vi "OCT with WavePond Clock.vi"() -> ()   [LabVIEW 2014]
doc: "I. Description:\nThis example demonstrates how to acquire a continuous amount of data (Waveform) using the DAQ device's internal clock.\n\nII. Instructions for Running:\n1. Create an analog input voltage channel.\n2. Set the rate for the sample clock. Additionally, define the sample mode to be continuous.\n3. Call the Start VI to start the acquisition.\n4. Read the waveform data in a loop until the user hits the stop button or an error occurs.\nNote: This example reads data from one or more channels and returns an array of data. Use the Index Array function to access an individual channel of data.\n5. Call the Clear Task VI to clear the Task.\n6. Use the popup dialog box to display an error if any.\n\nIV. I/O Connections Overview:\nMake sure your signal input terminal matches the Physical Channel I/O Control. For further connection information, refer to your hardware reference manual."
uses:
  ATS-VI/ATS_ctl/Device_Ctrl.ctl
  ATS-VI/ATS_ctl/ATS_Async_Ctrl.ctl
  ATS-VI/ATS_ctl/ATS_Async_Mode.ctl
  ATS-VI/ATS_ctl/ATS_DMA_Channel.ctl
  ATS-VI/ATS_ctl/ATS_ReadSamples.ctl
  ATS-VI/ATS_ctl/ATS_Check_Ctrl.ctl
  ATS-VI/ATS_ctl/ClockSource.ctl
  Galvo VIs/galvo_states.ctl
  Signal Processing/processing_states.ctl
  En Face/En Face States.ctl
  Saving Data/Saving Data States.ctl
  Type Defs/OCT Hardware States.ctl
  ATS-VI/ATS_ctl/Range.ctl
  ATS-VI/ATS_ctl/Impedance.ctl
  Type Defs/OCT Imaging Parameters Cluster.ctl
  Signal Processing/Display Raw Data states.ctl
  ATS-VI/ATS_ctl/ATS_Spec_Selector.ctl
  Classes/Galvo/Scanning Cluster.ctl
  Classes/Galvo/Galvo.lvclass
  Type Defs/OCT DAQ Channel Data Type.ctl
  Type Defs/Display States.ctl
  ATS-VI/ATS_ctl/Coupling.ctl
  ATS-VI/ATS_ctl/Bandwidth.ctl
  ATS-VI/ATS_ctl/InputCtrl.ctl
  ATS-VI/ATS_ctl/TriggerEngine.ctl
  ATS-VI/ATS_ctl/ExtTrigRange.ctl
  ATS-VI/ATS_ctl/ExtTrigger.ctl
  ATS-VI/ATS_ctl/TriggerOperation.ctl
  ATS-VI/ATS_ctl/Trigger.ctl
  ATS-VI/ATS_ctl/ClockRate.ctl
  ATS-VI/ATS_ctl/ClockEdge.ctl
  ATS-VI/ATS_ctl/Clock.ctl
  ATS-VI/ATS_ctl/Record.ctl
  ATS-VI/ATS_ctl/ATS_Global.ctl
  ATS-VI/ATS_ctl/ATS_Async_Status.ctl
  En Face/En Face Depth Parameters.ctl
  ATS-VI/ATS_ctl/ATS_Async_Setting.ctl
panel:
  in  "update en face image?":bool
  out "First Time?":bool
  out "Save Data":bool
  in  "Async_Setting":T1
  out "Processing Finished":bool
  in  "OCT Hardware States":T2=enum."Save Sweep"
  out "Save State":T3=enum."Initialize"
  out "Clock Length":u32=6304
  out "Reset DAQ":bool
  in  "Tab Control":T4(tab)
  in  "B-Scans Per Buffer":i32=1
  out "Async_Status":T5
  out "Current State":T2=enum."Set Resampling Array"
  in  "Channels":tag="Dev1/ao0:1"
  in  "Trigger Source":tag="/Dev1/PFI7"
  in  "Imaging Parameters":T6={"Points Per A-Scan"=0, "A-Scans per B-Scan"=0, "Voltage Range"=1.0, "Card Resolution (bits)"=12}
  in  "Setup_In":T7={"Record"={"Count"=1, "Presize"=0, "Length"=1408}, "Clock"={"ClckSource"=enum."External", "ClckRate"=17, "ClckEdge"=0, "Decimation"=0}, "Input A"={"Coupling"=enum."DC", "Range"=3, "Impedance"=enum."50 ohms", "Bandwidth"=enum."Full Bandwidth"}, "Input B"={"Coupling"=enum."DC", "Range"=3, "Impedance"=enum."50 ohms", "Bandwidth"=enum."Full Bandwidth"}, "Trigger"={"TrigOperation"=enum."Only X", "Timeout (s)"=1.0, "Trig. Delay"=0, "Engine X"={"Source"=enum."External", "Slope"=enum."Positive", "Level"=150}, "Engine Y"={"Source"=enum."Disable", "Slope"=enum."Positive", "Level"=128}, "ExtTrigControl"={"Coupling"=enum."DC", "Range"=enum."TTL"}}} {"Clock"."ClckEdge" items=["Rising", "Falling"]; "Clock"."ClckRate" items=["1 kS/s", "2 kS/s", "5 kS/s", "10 kS/s", "20 kS/s", "50 kS/s", "100 kS/s", "200 kS/s", "500 kS/s", "1 MS/s", "2 MS/s", "5 MS/s", "10 MS/s", "20 MS/s", "50 MS/s", "100 MS/s", "125 MS/s", "160 MS/s", "180 MS/s"]; "Input B"."Range" items=["200mV", "400mV", "800mV", "2 V", "4 V", "8 V", "16 V"]; "Trigger"."Timeout (s)" format="%.2f"; "Input A"."Range" items=["200mV", "400mV", "800mV", "2 V", "4 V", "8 V", "16 V"]}
  in  "OK Button":bool
  in  "Data Format":T23
  out "Channel A or B Phase (or Channel B Raw)":sgl[][](graph)
  out "Channel A or B Intensity (or Channel A Raw)":sgl[][](graph)
  in  "Display":T24
  out "En Face":dbl[][](graph)
  in  "En Face Parameters":T25={"En Face Start\nDepth"=50, "En Face End\nDepth"=200}
  in  "Save Sweep":bool
  in  "Scanning":T26={"Fast Axis Offset"=300.0, "Slow Axis Offset"=300.0, "Slow Axis Amp"=4.0, "Fast Axis Amp"=4.0, "Scan Pattern"=enum."Raster"} {"Fast Axis Amp" max=20 format="%#.2f"; "Slow Axis Amp" max=20 format="%#.2f"; "Slow Axis Offset" max=10 format="%#.2f"; "Fast Axis Offset" max=10 format="%#.2f"}
  in  "Stop Button":bool
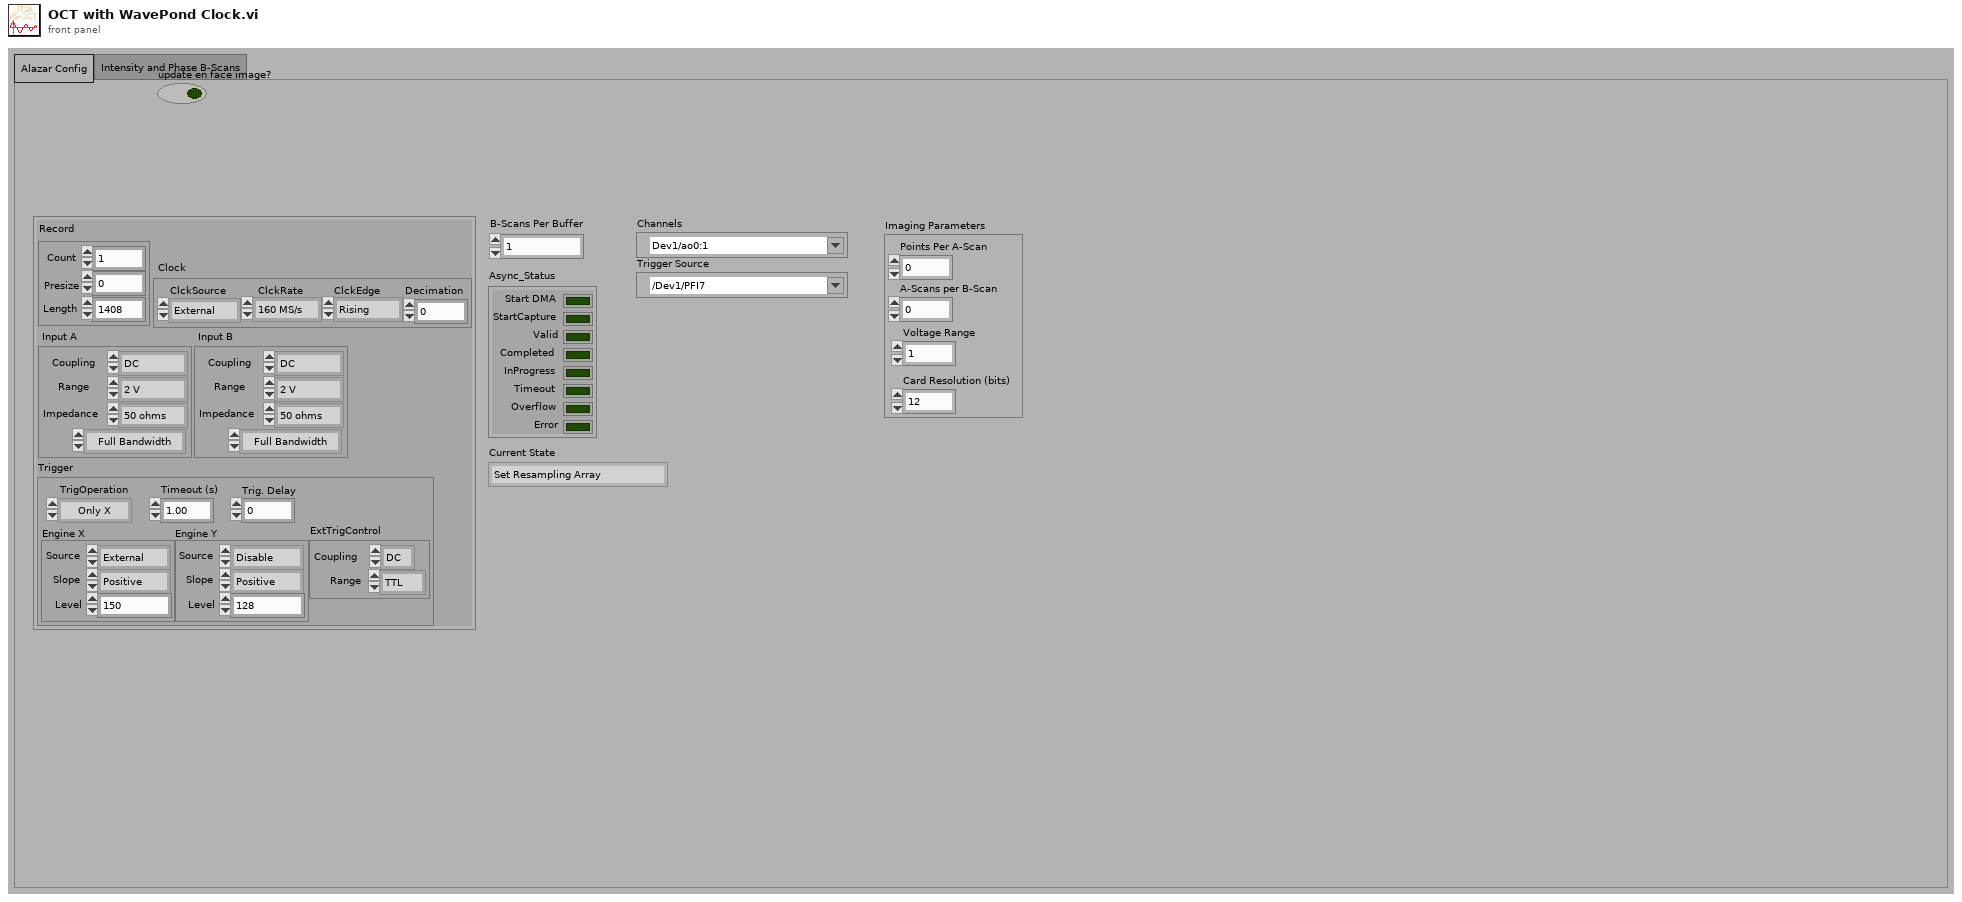
[diagram p1: front panel]
types:
  T1 = typedef "ATS_Async_Setting.ctl" = cluster{"UseHeader":u32, "Rec/Buffer":u32, "Total_Rec":u32, "DataBuffer":bool, "GetProcessedData":bool}
  T2 = typedef "OCT Hardware States.ctl" = enum16{"Acquire Data", "Initialize Laser", "Initialize Galvos", "Startup", "Reset DAQ", "Background Subtraction", "Acquire Background", "Update DAQ Parameters", "Stop", "Set Clock", "Initialize DAQ", "Set Resampling Array", "Save Sweep", "Configure Laser", "128 x 128", "512 x 512", "Review Data"}
  T3 = typedef "Saving Data States.ctl" = enum16{"Get Queue Size", "Get Queue", "Get Timeout", "Flush Queue", "Close Files", "Create Files", "Do Nothing", "Initialize", "Enqueue Data", "Save Data", "Shutdown"}
  T4 = enum32{"Alazar Config", "Intensity and Phase B-Scans"}
  T5 = typedef "ATS_Async_Status.ctl" = cluster{"Start DMA":bool, "StartCapture":bool, "Valid":bool, "Completed":bool, "InProgress":bool, "Timeout":bool, "Overflow":bool, "Error":bool}
  T6 = typedef "OCT Imaging Parameters Cluster.ctl" = cluster{"Points Per A-Scan":i32, "A-Scans per B-Scan":i32, "Voltage Range":sgl, "Card Resolution (bits)":u16}
  T7 = typedef "ATS_Global.ctl" = cluster{"Record":T8, "Clock":T9, "Input A":T13, "Input B":T13, "Trigger":T18}
  T8 = typedef "Record.ctl" = cluster{"Count":u32, "Presize":u32, "Length":u32}
  T9 = typedef "Clock.ctl" = cluster{"ClckSource":T10, "ClckRate":T11, "ClckEdge":T12, "Decimation":u32}
  T10 = typedef "ClockSource.ctl" = enum16{"Internal", "External", "Medium Ext.", "Slow Ext.", "Ext. AC", "Ext. DC", "Ext. (PLL)"}
  T11 = typedef "ClockRate.ctl" = u32
  T12 = typedef "ClockEdge.ctl" = u16
  T13 = typedef "InputCtrl.ctl" = cluster{"Coupling":T14, "Range":T15, "Impedance":T16, "Bandwidth":T17}
  T14 = typedef "Coupling.ctl" = enum16{"AC", "DC"}
  T15 = typedef "Range.ctl" = u32
  T16 = typedef "Impedance.ctl" = enum16{"1M ohms", "50 ohms"}
  T17 = typedef "Bandwidth.ctl" = enum16{"Full Bandwidth", "Reduce Bandwidth"}
  T18 = typedef "Trigger.ctl" = cluster{"TrigOperation":T19, "Timeout (s)":dbl, "Trig. Delay":u32, "Engine X":T20, "Engine Y":T20, "ExtTrigControl":T21}
  T19 = typedef "TriggerOperation.ctl" = enum16{"Only X", "Only Y", "X or Y", "X and Y", "X xor Y", "X and not Y", "not X and Y"}
  T20 = typedef "TriggerEngine.ctl" = cluster{"Source":enum32{"Chan_A", "Chan_B", "External", "Disable"}, "Slope":enum32{"Positive", "Negative"}, "Level":u32}
  T21 = typedef "ExtTrigger.ctl" = cluster{"Coupling":T14, "Range":T22}
  T22 = typedef "ExtTrigRange.ctl" = enum16{"1 V", "5 V", "TTL"}
  T23 = typedef "OCT DAQ Channel Data Type.ctl" = enum16{"Channel 1", "Channel 2", "Channel 1 and 2"}
  T24 = typedef "Display States.ctl" = enum16{"Channel A", "Channel B"}
  T25 = typedef "En Face Depth Parameters.ctl" = cluster{"En Face Start\nDepth":i32, "En Face End\nDepth":i32}
  T26 = typedef "Galvo.lvclass/Scanning Cluster.ctl" = cluster{"Fast Axis Offset":sgl, "Slow Axis Offset":sgl, "Slow Axis Amp":sgl, "Fast Axis Amp":sgl, "Scan Pattern":enum16{"Raster"}}
  T27 = typedef "ATS_Check_Ctrl.ctl" = enum16{"None", "NO_ATS9462", "ATS9462_Traditional", "Verify Board", "OnBoard Memory", "Board & Memory", "Master/Slave", "NO Master/Slave"}
  T28 = typedef "Device_Ctrl.ctl" = enum16{"Status", "About", "Arm", "ForceTrig", "Abort", "Initialize", "Init (NoPreset)", "Info", "Close", "Calibrate", "SetManually", "LED_ON", "LED_OFF"}
  T29 = typedef "ATS_Spec_Selector.ctl" = enum16{"None", "ClckSource", "ClckEdge", "ClckRate", "InputRange", "InputCoupling", "Impedance", "Bandwidth", "AsyncDMA", "Memory", "ExtTrigCoupling", "ExtTrigRange", "AUX_IO_Trig", "AUX_IO_Slope", "Trigger_Source"}
  T30 = typedef "galvo_states.ctl" = enum16{"Reset", "Reset Galvos?", "Center Galvos", "Register Callback", "Get Scan Parameters", "Show", "Initialize", "Run Raster", "Load Raster", "Run Circle", "Shutdown"}
  T31 = typedef "processing_states.ctl" = enum16{"Initialize", "Set Background", "Update Imaging Parameters", "Get Queue", "Process Data", "Get Size", "Flush Data", "Set Reample Array", "Get Last Processed BScan", "Shutdown"}
  T32 = typedef "Display Raw Data states.ctl" = enum16{"Add Raw", "Add Processed", "Show"}
  T33 = typedef "En Face States.ctl" = enum16{"Save BMP", "Show", "Clear En Face", "Update EnFace"}
  T34 = typedef "Processed OCT Data.ctl" = cluster{"Intensity A":sgl[][][], "Phase A":sgl[][][], "Intensity B":sgl[][][], "Phase B":sgl[][][]}
  T35 = enum8{"Enabled", "Disabled", "Disabled and Grayed Out"}
  T36 = typedef "ATS_Async_Ctrl.ctl" = enum16{"SetupDMA", "StartCapture", "Get", "Get_Stream", "Abort", "Stop"}
  T37 = typedef "ATS_ReadSamples.ctl" = cluster{"Offset":i32, "Length":u32}
  T38 = typedef "ATS_DMA_Channel.ctl" = enum16{"Channel_A", "Channel_B", "A & B"}
  T39 = typedef "ATS_Async_Mode.ctl" = enum16{"Continuous", "Triggered", "No-Pre-Trigger", "Traditional"}
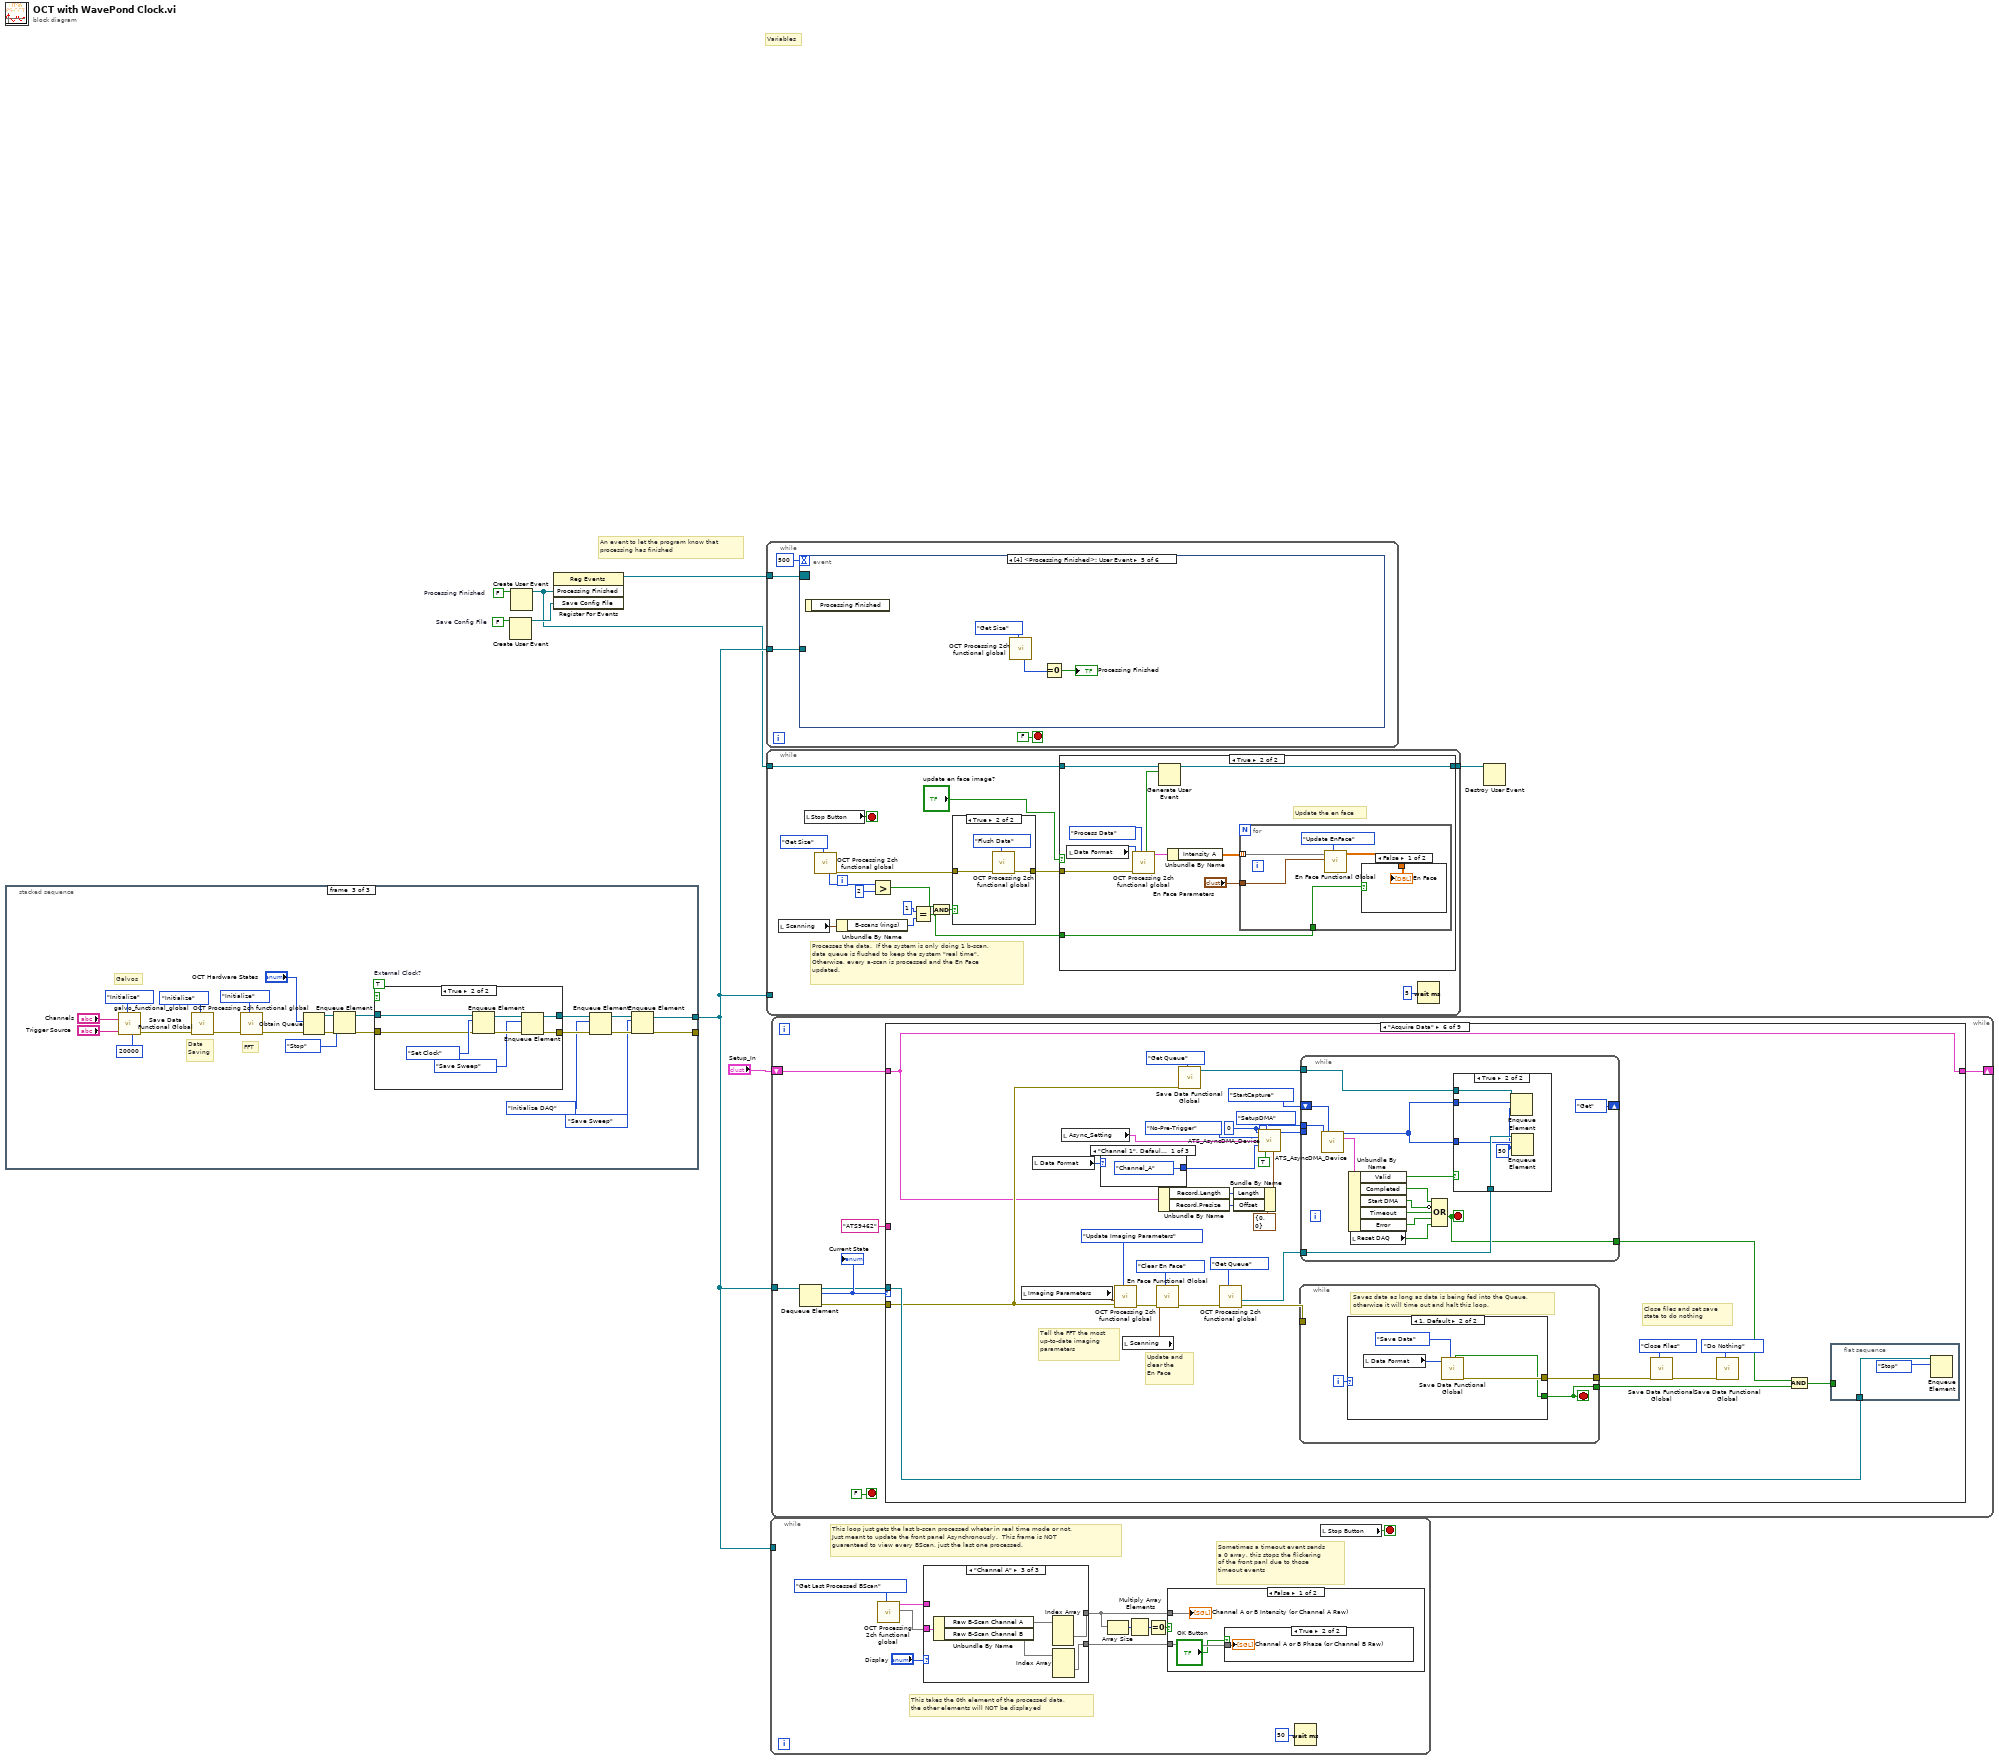
[diagram p0: block diagram]
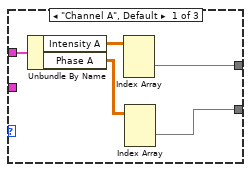
[diagram p7: hidden frame]
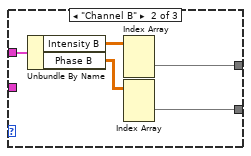
[diagram p8: hidden frame]
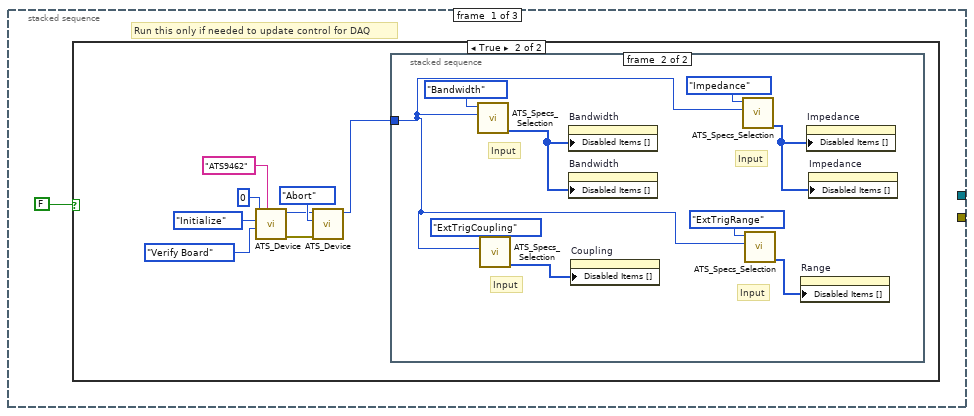
[diagram p9: hidden frame]
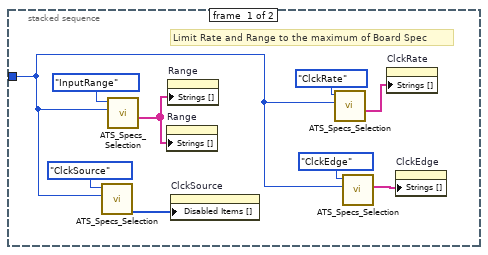
[diagram p11: hidden frame]
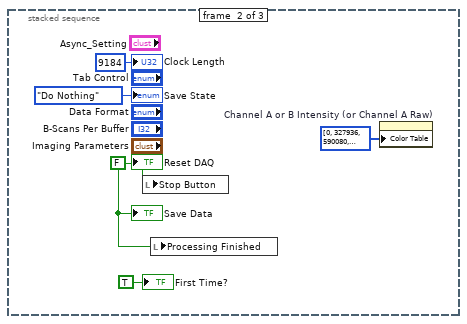
[diagram p12: hidden frame]
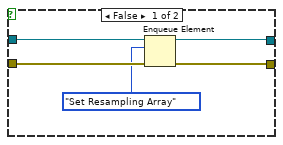
[diagram p13: hidden frame]
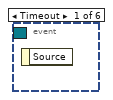
[diagram p14: hidden frame]
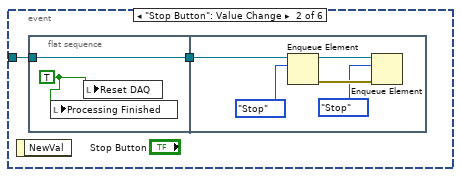
[diagram p15: hidden frame]
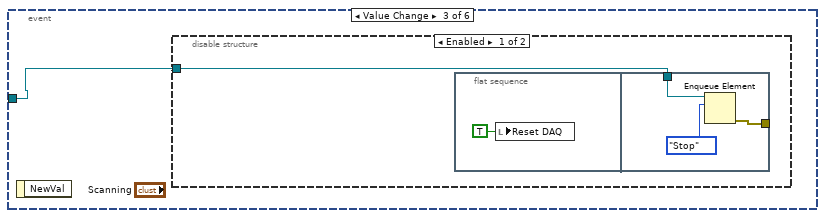
[diagram p16: hidden frame]
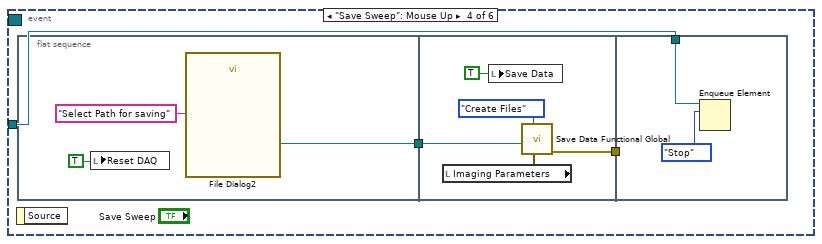
[diagram p18: hidden frame]
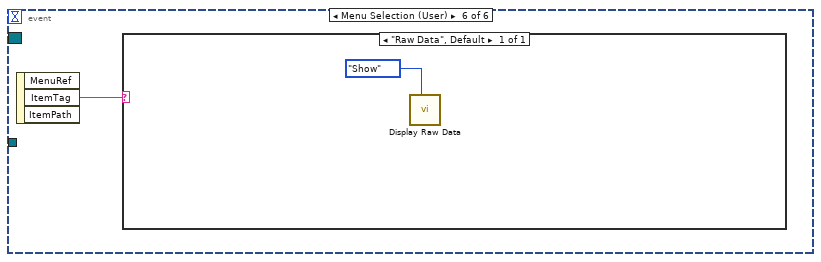
[diagram p19: hidden frame]
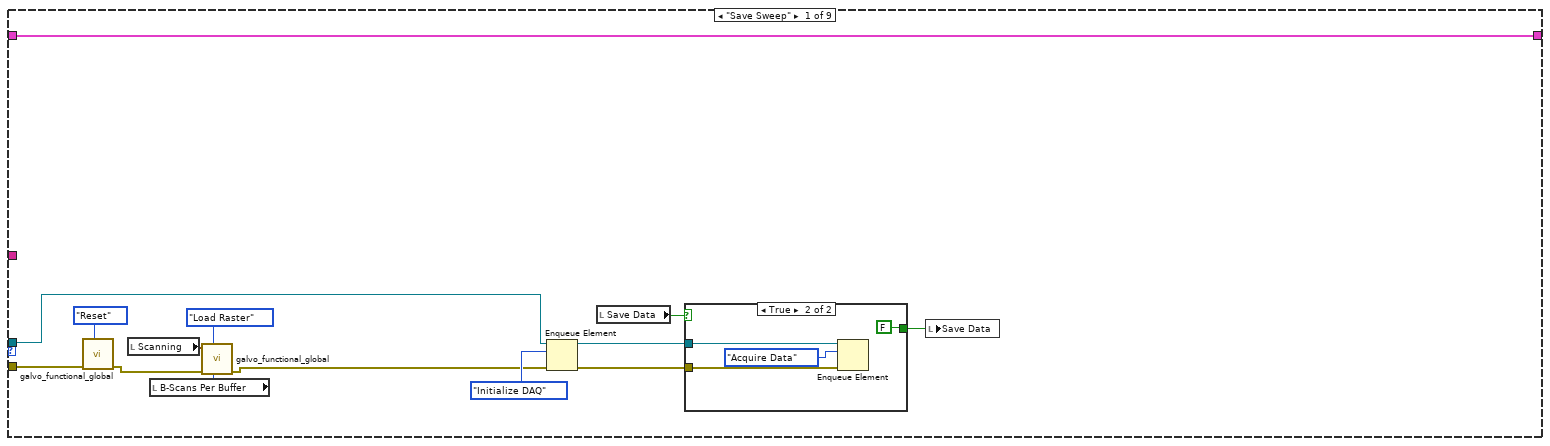
[diagram p20: hidden frame]
diagram:
  w1 = FALSE  # Save Config File
  w8 = FALSE  # Processing Finished
  # "An event to let the program know that\nprocessing has finished"
  # "Variables"
  n1 = stacked-sequence {
    tunnel: [_ _ w54] -> _
    tunnel: [_ _ w60] -> w5
    frame #0 {
      # "Run this only if needed to update control for DAQ"
      n2 = case shown="True" FALSE {
        frame False {
        }
        frame True {
          n3 = call "ATS_Device.vi"("BoardToVerify"="ATS9462", "ATS_Check"=ATS_Check_Ctrl."Verify Board", "DevCtrl"=Device_Ctrl."Initialize", "DeviceIn"=0 ("Device")) -> ("error out"=w13:errorcluster, "DeviceOut"=w15:i32)  [unwired: 1 in, 5 out]
          n4 = call "ATS_Device.vi"("error in (no error)"=w13, "DevCtrl"=Device_Ctrl."Abort", "DeviceIn"=w15) -> ("DeviceOut"=w11:i32)  [unwired: 2 in, 6 out]
          n5 = stacked-sequence {
            tunnel: w11 -> [w20 w27]
            frame #0 {
              # "Limit Rate and Range to the maximum of Board Spec"
              n6 = call "ATS_Specs_Selection.vi"("Device"=w20, "ATS_Spec_Selector"=ATS_Spec_Selector."ClckSource") -> ("Disabled_Item"=w19:i32[])  [unwired: 3 in, 6 out]
              n7 = call "ATS_Specs_Selection.vi"("Device"=w20, "ATS_Spec_Selector"=ATS_Spec_Selector."InputRange") -> ("Possible_Item"=w26:string[])  [unwired: 3 in, 6 out]
              n8 = property on="Range" class="Ring (strict)"("Strings []"=w26) -> ()  [unwired: 2 in, 2 out]
              n9 = property on="Range" class="Ring (strict)"("Strings []"=w26) -> ()  [unwired: 2 in, 2 out]
              n10 = property on="ClckSource" class="Enum (strict)"("Disabled Items []"=w19) -> ()  [unwired: 2 in, 2 out]
              n11 = call "ATS_Specs_Selection.vi"("Device"=w20, "ATS_Spec_Selector"=ATS_Spec_Selector."ClckRate") -> ("Possible_Item"=w24:string[])  [unwired: 3 in, 6 out]
              n12 = call "ATS_Specs_Selection.vi"("Device"=w20, "ATS_Spec_Selector"=ATS_Spec_Selector."ClckEdge") -> ("All_Item"=w18:string[])  [unwired: 3 in, 6 out]
              n13 = property on="ClckRate" class="Ring (strict)"("Strings []"=w24) -> ()  [unwired: 2 in, 2 out]
              n14 = property on="ClckEdge" class="Ring (strict)"("Strings []"=w18) -> ()  [unwired: 2 in, 2 out]
            }
            frame #1 {
              # "Input"
              # "Input"
              # "Input"
              # "Input"
              n15 = call "ATS_Specs_Selection.vi"("Device"=w27, "ATS_Spec_Selector"=ATS_Spec_Selector."Bandwidth") -> ("Disabled_Item"=w33:i32[])  [unwired: 3 in, 6 out]
              n16 = call "ATS_Specs_Selection.vi"("Device"=w27, "ATS_Spec_Selector"=ATS_Spec_Selector."ExtTrigCoupling") -> ("Disabled_Item"=w29:i32[])  [unwired: 3 in, 6 out]
              n17 = property on="Bandwidth" class="Enum (strict)"("Disabled Items []"=w33) -> ()  [unwired: 2 in, 2 out]
              n18 = property on="Bandwidth" class="Enum (strict)"("Disabled Items []"=w33) -> ()  [unwired: 2 in, 2 out]
              n19 = property on="Coupling" class="Enum (strict)"("Disabled Items []"=w29) -> ()  [unwired: 2 in, 2 out]
              n20 = call "ATS_Specs_Selection.vi"("Device"=w27, "ATS_Spec_Selector"=ATS_Spec_Selector."Impedance") -> ("Disabled_Item"=w32:i32[])  [unwired: 3 in, 6 out]
              n21 = call "ATS_Specs_Selection.vi"("Device"=w27, "ATS_Spec_Selector"=ATS_Spec_Selector."ExtTrigRange") -> ("Disabled_Item"=w28:i32[])  [unwired: 3 in, 6 out]
              n22 = property on="Range" class="Enum (strict)"("Disabled Items []"=w28) -> ()  [unwired: 2 in, 2 out]
              n23 = property on="Impedance" class="Enum (strict)"("Disabled Items []"=w32) -> ()  [unwired: 2 in, 2 out]
              n24 = property on="Impedance" class="Enum (strict)"("Disabled Items []"=w32) -> ()  [unwired: 2 in, 2 out]
            }
          }
        }
      }
    }
    frame #1 {
      w37 = FALSE ("Sweep Ready for saving")
      n25 = local write "Stop Button"(w37) -> ()
      n26 = local write "Processing Finished"(w37) -> ()
      n27 = property on="Channel A or B Intensity (or Channel A Raw)" class="IntGraph (strict)"("Color Table"=u32[] [0, 327936, 590080, 852224, 983296, 1114624, 1180160, 1311232, 1442304, 1573632, 1704704, 1770240, 1901312, 1966848, 2098176, 2163712, 2294784, 2491392, 2557184, 2688256, 2753792, 2884864, 2950656, 3081728, 3147264, 3344129, 3475457, 3540993, 3672321, 3738113, 3869185, 3934977, 4066305, 4197633, 4328961, 4394497, 4460289, 4591617, 4657409, 4788481, 4854273, 4985601, 5116929, 5248257, 5314049, 5379841, 5511169, 5576961, 5708033, 5773825, 5905153, 6036482, 6167810, 6233346, 6299138, 6430466, 6496258, 6562050, 6693634, 6759426, 6890754, 7022082, 7087874, 7153666, 7284994, 7350786, 7482114, 7547906, 7613698, 7745026, 7876354, 8007682, 8073474, 8139522, 8205314, 8336642, 8467970, 8533763, 8599555, 8665347, 8731139, 8862467, 8993795, 9059587, 9125380, 9191428, 9257220, 9388548, 9454340, 9520132, 9585924, 9717253, 9848837, 9914629, 9980165, 10045957, 10177541, 10243334, 10309126, 10375174, 10440966, 10572294, 10703623, 10769416, 10835208, 10901256, 10967049, 11033097, 11033609, 11099401, 11165450, 11231242, 11231754, 11297547, 11363339, 11429131, 11495180, 11495692, 11561740, 11693069, 11758861, 11759373, 11825165, 11891214, 11957006, 12022799, 12023311, 12089103, 12220944, 12286736, 12286736, 12352529, 12418577, 12484370, 12550162, 12615954, 12681747, 12747796, 12813588, 12813845, 12879894, 12945686, 13077015, 13142808, 13143064, 13208856, 13274905, 13340697, 13340953, 13472282, 13538075, 13604379, 13670172, 13735964, 13801757, 13867550, 13933343, 13999392, 13999648, 14065441, 14131234, 14197027, 14197541, 14263334, 14329383, 14395176, 14460969, 14592553, 14658346, 14724139, 14789932, 14790189, 14856238, 14922287, 14988080, 15053873, 15054130, 15119923, 15185972, 15251765, 15317559, 15383353, 15449146, 15449660, 15515454, 15515968, 15516226, 15582021, 15582278, 15582536, 15648587, 15648844, 15714639, 15714897, 15715155, 15780949, 15781463, 15847256, 15847770, 15848028, 15913823, 15914081, 15979875, 15980133, 15980391, 16046441, 16046444, 16046703, 16046705, 16112500, 16113015, 16113274, 16113277, 16179072, 16179330, 16179588, 16245384, 16245387, 16245389, 16245648, 16311443, 16376982, 16377241, 16377499, 16443294, 16443553, 16443555, 16443815, 16509866, 16510124, 16510127, 16575923, 16575924, 16576182, 16576441, 16576443, 16576702, 16576705, 16576963, 16577222, 16577224, 16577482, 16577485, 16577743, 16577745, 16578004, 16578262, 16578264, 16578523, 16578782, 16579040, 16579299, 16579301, 16579303, 16579562, 16579821]) -> ()  [unwired: 2 in, 2 out]
      "Clock Length" <- u32 9184 ("Clock Length")
      "Save State" <- Saving_Data_States."Do Nothing" ("Save State")
      "Reset DAQ" <- w37
      "Save Data" <- w37
      "First Time?" <- TRUE ("First Time?")
    }
    frame #2 {
      w42 = TRUE  # External Clock?
      # "FFT"
      # "Data \nSaving"
      # "Galvos"
      n28 = call "galvo_functional_global.vi"(4:20000 ("Sweep Speed"), "State"=galvo_states."Initialize", "Trigger Source"="Trigger Source", "Analog Output"="Channels") -> ("error out"=w51:errorcluster)  [unwired: 6 in, 1 out]
      n29 = call "Save Data Functional Global.vi"("States"=Saving_Data_States."Initialize", "error in (no error)"=w51) -> ("error out"=w56:errorcluster)  [unwired: 6 in, 3 out]
      n30 = call "OCT Processing 2ch functional global.vi"("State"=processing_states."Initialize", "error in (no error)"=w56) -> ("error out"=w57:errorcluster)  [unwired: 5 in, 4 out]
      n31 = Obtain Queue(element data type="OCT Hardware States", error in (no error)=w57) -> (queue out=w45:refnum<queue>, error out=w44:errorcluster)  [unwired: 3 in, 1 out]
      n32 = Enqueue Element(queue=w45, element=OCT_Hardware_States."Stop", error in (no error)=w44) -> (queue out=w47:refnum<queue>, error out=w46:errorcluster)  [unwired: 1 in, 1 out]
      n33 = case shown="True" w42 {
        tunnel: [w66 w75] -> w64
        tunnel: [w67 w74] -> w63
        tunnel: w47 -> [w69 w71]
        tunnel: w46 -> [w68 w70]
        frame False {
          n34 = Enqueue Element(queue=w69, element=OCT_Hardware_States."Set Resampling Array", error in (no error)=w68) -> (queue out=w66:refnum<queue>, error out=w67:errorcluster)  [unwired: 1 in, 1 out]
        }
        frame True {
          n35 = Enqueue Element(queue=w71, element=OCT_Hardware_States."Set Clock", error in (no error)=w70) -> (queue out=w77:refnum<queue>, error out=w76:errorcluster)  [unwired: 1 in, 1 out]
          n36 = Enqueue Element(queue=w77, element=OCT_Hardware_States."Save Sweep", error in (no error)=w76) -> (queue out=w75:refnum<queue>, error out=w74:errorcluster)  [unwired: 1 in, 1 out]
        }
      }
      n37 = Enqueue Element(queue=w64, element=OCT_Hardware_States."Initialize DAQ", error in (no error)=w63) -> (queue out=w62:refnum<queue>, error out=w61:errorcluster)  [unwired: 1 in, 1 out]
      n38 = Enqueue Element(queue=w62, element=OCT_Hardware_States."Save Sweep", error in (no error)=w61) -> (queue out=w60:refnum<queue>, error out=w54:errorcluster)  [unwired: 1 in, 1 out]
    }
  }
  n39 = Create User Event(user event datatype=w1) -> (user event=w4:refnum<user-event>)  [unwired: 1 in, 1 out]
  n40 = Create User Event(user event datatype=w8) -> (user event=w3:refnum<user-event>)  [unwired: 1 in, 1 out]
  n41 = register-events(w3, w4) -> (reference out=w7:refnum<event-registration>)  [unwired: 2 in, 1 out]
  n42 = while {
    tunnel: w5 -> [w79]
    tunnel: w7 -> [w80]
    stop <- FALSE stop-if-true
    n43 = event shown="[4] <Processing Finished>: User Event" {
      selector: w80 -> [_ _ _ _ _ _]
      dyn-events: _ -> [_ _ _ _ _ _]
      timeout: 500 -> [_ _ _ _ _ _]
      tunnel: w79 -> [_ w82 w91 w99 _ _]
      event Timeout {
        n44 = event-data() -> ()  [unwired: 1 in, 1 out]
      }
      event "Stop Button": Value Change {
        n45 = event-data() -> ()  [unwired: 1 in, 1 out]
        n46 = flat-sequence {
          tunnel: w82 -> [w85]
          tunnel: [w85] -> w83
          tunnel: w83 -> [w90]
          frame #0 {
            w84 = TRUE ("Reset DAQ")
            n47 = local write "Processing Finished"(w84) -> ()
            n48 = local write "Reset DAQ"(w84) -> ()
          }
          frame #1 {
            n49 = Enqueue Element(queue=w90, element=OCT_Hardware_States."Stop") -> (queue out=w87:refnum<queue>, error out=w88:errorcluster)  [unwired: 2 in, 1 out]
            n50 = Enqueue Element(queue=w87, element=OCT_Hardware_States."Stop", error in (no error)=w88) -> ()  [unwired: 1 in, 3 out]
          }
        }
      }
      event Value Change {
        n51 = event-data() -> ()  [unwired: 1 in, 1 out]
        n52 = disable-structure shown="Enabled" {
          disable-tunnel: w91 -> [w92 _]
          frame Enabled {
            n53 = flat-sequence {
              tunnel: w92 -> [w95]
              tunnel: [w94] -> _
              frame #0 {
                n54 = local write "Reset DAQ"(TRUE ("Reset DAQ")) -> ()
              }
              frame #1 {
                n55 = Enqueue Element(queue=w95, element=OCT_Hardware_States."Stop") -> (error out=w94:errorcluster)  [unwired: 2 in, 2 out]
              }
            }
          }
          frame Disabled {
          }
        }
      }
      event "Save Sweep": Mouse Up {
        n56 = event-data() -> ()  [unwired: 1 in, 1 out]
        n57 = flat-sequence {
          tunnel: [w100] -> w98
          tunnel: w98 -> [w107]
          tunnel: [w105] -> w97
          tunnel: w99 -> [w109]
          tunnel: w97 -> [_]
          frame #0 {
            n58 = local write "Reset DAQ"(TRUE ("Reset DAQ")) -> ()
            n59 = call "File Dialog2"("prompt"="Select Path for saving") -> ("selected path"=w100:path)  [unwired: 11 in, 3 out]
          }
          frame #1 {
            n60 = local read "Imaging Parameters"() -> (w104:T6)
            n61 = local write "Save Data"(TRUE ("Save Data")) -> ()
            n62 = call "Save Data Functional Global.vi"("Input Parameters"=w104, "States"=Saving_Data_States."Create Files", "Folder"=w107) -> ("error out"=w105:errorcluster)  [unwired: 5 in, 3 out]
          }
          frame #2 {
            n63 = Enqueue Element(queue=w109, element=OCT_Hardware_States."Stop") -> ()  [unwired: 2 in, 3 out]
          }
        }
      }
      event User Event {
        n64 = event-data() -> ()  [unwired: 1 in, 1 out]
        n65 = call "OCT Processing 2ch functional global.vi"("State"=processing_states."Get Size") -> ("# elements in queue"=w111:i32)  [unwired: 6 in, 4 out]
        n66 = Equal To 0?(x=w111) -> (x = 0?=→"Processing Finished":bool)
      }
      event Menu Selection (User) {
        n67 = event-data() -> ("ItemTag"=w113:string)  [unwired: 1 in, 2 out]
        n68 = case shown="\"Raw Data\", Default" w113 {
          frame "Raw Data", Default {
            n69 = call "Display Raw Data.vi"("Enum"=Display_Raw_Data_states."Show") -> ()  [unwired: 11 in]
          }
        }
      }
    }
  }
  n70 = while {
    tunnel: w3 -> [w121]
    tunnel: [w120] -> w6
    tunnel: w5 -> [_]
    stop <- w130 stop-if-true
    # "Processes the data.  If the system is only doing 1 b-scan, \ndata queue is flushed to keep the system \"real time\".\nOtherwise, every a-scan is processed and the En Face\nupdated."
    n71 = local read "Scanning"() -> (w123:T26)
    n72 = local read "Stop Button"() -> (w130:bool)
    n73 = call "OCT Processing 2ch functional global.vi"("State"=processing_states."Get Size") -> ("error out"=w119:errorcluster, "# elements in queue"=w127:i32)  [unwired: 6 in, 3 out]
    n74 = Unbundle By Name(w123) -> ("B-scans (rings)"=w122:u32)
    n75 = Greater?(x=w127, y=2) -> (0:w128:bool)
    n76 = Equal?(x=u32 1, y=w122) -> (x = y?=w116:bool)
    n77 = And(x=w128, y=w116) -> (x .and. y?=w117:bool)
    n78 = case shown="True" w117 {
      tunnel: w119 -> [w148 w151]
      tunnel: [w148 w150] -> w118
      frame False {
      }
      frame True {
        n79 = call "OCT Processing 2ch functional global.vi"("State"=processing_states."Flush Data", "error in (no error)"=w151) -> ("error out"=w150:errorcluster)  [unwired: 5 in, 4 out]
      }
    }
    n80 = case shown="True" "update en face image?" {
      tunnel: w121 -> [w131 w138]
      tunnel: [w131 w136] -> w120
      tunnel: w118 -> [_ w133]
      tunnel: w116 -> [_ w132]
      frame False {
      }
      frame True {
        # "Update the en face"
        n81 = local read "Data Format"() -> (w139:T23)
        n82 = call "OCT Processing 2ch functional global.vi"("State"=processing_states."Process Data", "error in (no error)"=w133, "Data Format"=w139) -> ("Processed OCT Data"=w140:T34, "Time Out"=w137:bool)  [unwired: 4 in, 3 out]
        n83 = Generate User Event(user event=w138, event data cluster=w137) -> (user event out=w136:refnum<user-event>)  [unwired: 2 in, 1 out]
        n84 = Unbundle By Name(w140) -> ("Intensity A"=w134:sgl[][][])
        n85 = for {
          tunnel: "En Face Parameters" -> [w145]
          tunnel: w134 -> [w144] mode=indexing
          tunnel: w132 -> [w142]
          n86 = call "En Face Functional Global.vi"(7:En_Face_States."Update EnFace" ("En Face States"), 10:w145, "Intensity Graph 2"=w144) -> ("Intensity Graph"=w143:dbl[][])  [unwired: 7 in, 1 out]
          n87 = case shown="False" w142 {
            tunnel: w143 -> [w147 _]
            frame False {
              "En Face" <- w147
            }
            frame True {
            }
          }
        }
      }
    }
    n88 = Wait (ms)(milliseconds to wait=u32 5) -> ()  [unwired: 1 out]
  }
  n89 = while {
    tunnel: w5 -> [_]
    stop <- w162 stop-if-true
    # "Sometimes a timeout event sends\na 0 array, this stops the flickering\nof the front panl due to those \ntimeout events"
    # "This takes the 0th element of the processed data,\nthe other elements will NOT be displayed"
    # "This loop just gets the last b-scan processed wheter in real time mode or not. \nJust meant to update the front panel Asynchronously.  This frame is NOT\nguarenteed to view every BScan, just the last one processed."
    n90 = call "OCT Processing 2ch functional global.vi"("State"=processing_states."Get Last Processed BScan") -> (2:w158, "Processed OCT Data"=w156:T34)  [unwired: 5 in, 4 out]
    n91 = case shown="\"Raw Data A and B\"" "Display" {
      tunnel: w156 -> [w171 w172 _]
      tunnel: w158 -> [_ _ w181]
      tunnel: [w167 w174 w179] -> w154
      tunnel: [w168 w173 w178] -> w157
      frame "Channel A", Default {
        n92 = Unbundle By Name(w171) -> ("Intensity A"=w169:sgl[][][], "Phase A"=w170:sgl[][][])
        n93 = Index Array(array=w169) -> (element=w167:sgl[][])  [unwired: 3 in]
        n94 = Index Array(array=w170) -> (element=w168:sgl[][])  [unwired: 3 in]
      }
      frame "Channel B" {
        n95 = Unbundle By Name(w172) -> ("Intensity B"=w175:sgl[][][], "Phase B"=w176:sgl[][][])
        n96 = Index Array(array=w175) -> (element=w174:sgl[][])  [unwired: 3 in]
        n97 = Index Array(array=w176) -> (element=w173:sgl[][])  [unwired: 3 in]
      }
      frame "Channel A" {
        n98 = Unbundle By Name(w181) -> ("Raw B-Scan Channel A"=w177, "Raw B-Scan Channel B"=w180)
        n99 = Index Array(array=w177) -> (element=w179)  [unwired: 3 in]
        n100 = Index Array(array=w180) -> (element=w178)  [unwired: 3 in]
      }
    }
    n101 = Array Size(array=w154) -> (size(s)=w155:i32[])
    n102 = Multiply Array Elements(1:w155) -> (0:w153:i32)
    n103 = Equal To 0?(x=w153) -> (x = 0?=w152:bool)
    n104 = case shown="False" w152 {
      tunnel: w157 -> [w165 _]
      tunnel: w154 -> [w164 _]
      frame False {
        n105 = case shown="True" "OK Button" {
          tunnel: w165 -> [_ w166]
          frame False {
          }
          frame True {
            "Channel A or B Phase (or Channel B Raw)" <- w166
          }
        }
        "Channel A or B Intensity (or Channel A Raw)" <- w164
      }
      frame True {
      }
    }
    n106 = Wait (ms)(milliseconds to wait=u32 50) -> ()  [unwired: 1 out]
    n107 = local read "Stop Button"() -> (w162:bool)
  }
  n108 = while {
    tunnel: w5 -> [w189]
    shift-right: [w183] -> _
    shift-left: "Setup_In" -> [w182]
    stop <- FALSE stop-if-true
    n109 = Dequeue Element(queue=w189) -> (queue out=w185:refnum<queue>, element=w187:T2, error out=w186:errorcluster)  [unwired: 2 in, 1 out]
    "Current State" <- w187
    n110 = case shown="\"Acquire Data\"" w187 {
      tunnel: w186 -> [w203 w218 _ _ w320 w376 _ w448 _]
      tunnel: w185 -> [w202 w220 _ _ w329 w391 _ w449 _]
      tunnel: "ATS9462" ("BoardToVerify") -> [_ _ _ w281 _ _ _ _ w456]
      tunnel: [w201 w215 w231 w275 w316 w374 w438 w440 w455] -> w183
      tunnel: w182 -> [w201 w215 w231 w274 w316 w374 w438 w440 w455]
      frame "Save Sweep" {
        n111 = call "galvo_functional_global.vi"("State"=galvo_states."Reset", "error in (no error)"=w203) -> ("error out"=w191:errorcluster)  [unwired: 8 in, 1 out]
        n112 = local read "Scanning"() -> (w193:T26)
        n113 = local read "B-Scans Per Buffer"() -> (w194:i32)
        n114 = call "galvo_functional_global.vi"("Est Sweep Speed"=w194, "State"=galvo_states."Load Raster", "error in (no error)"=w191, "user event out"=w193) -> ("error out"=w190:errorcluster)  [unwired: 6 in, 1 out]
        n115 = Enqueue Element(queue=w202, element=OCT_Hardware_States."Initialize DAQ", error in (no error)=w190) -> (queue out=w199:refnum<queue>, error out=w198:errorcluster)  [unwired: 1 in, 1 out]
        n116 = local read "Save Data"() -> (w197:bool)
        n117 = case shown="True" w197 {
          tunnel: w199 -> [w206 w211]
          tunnel: w198 -> [w205 w210]
          tunnel: [FALSE ("Reset DAQ") FALSE ("Reset DAQ")] -> w196
          frame False {
            n118 = Enqueue Element(queue=w206, element=OCT_Hardware_States."Acquire Data", error in (no error)=w205) -> ()  [unwired: 1 in, 3 out]
          }
          frame True {
            n119 = Enqueue Element(queue=w211, element=OCT_Hardware_States."Acquire Data", error in (no error)=w210) -> ()  [unwired: 1 in, 3 out]
          }
        }
        n120 = local write "Save Data"(w196) -> ()
      }
      frame "Stop" {
        n121 = flat-sequence {
          tunnel: w218 -> [w229]
          tunnel: [w229] -> w217
          frame #0 {
            n122 = local write "Processing Finished"(FALSE ("Reset DAQ")) -> ()
            n123 = local write "Reset DAQ"(FALSE ("Reset DAQ")) -> ()
          }
        }
        n124 = call "Save Data Functional Global.vi"("States"=Saving_Data_States."Flush Queue", "error in (no error)"=w217) -> ("error out"=w222:errorcluster)  [unwired: 6 in, 3 out]
        n125 = call "OCT Processing 2ch functional global.vi"("State"=processing_states."Flush Data", "error in (no error)"=w222) -> ("error out"=w214:errorcluster)  [unwired: 5 in, 4 out]
        n126 = property on="Save Sweep" class="Bool"(error in=w214, "DisabledEnum"=T35."Disabled and Grayed Out" ("Disabled")) -> (error out=w213:errorcluster)  [unwired: 1 in, 1 out]
        n127 = Enqueue Element(queue=w220, element=OCT_Hardware_States."Save Sweep", error in (no error)=w213) -> (error out=w216:errorcluster)  [unwired: 1 in, 2 out]
        n128 = flat-sequence {
          tunnel: w216 -> [_]
          frame #0 {
            w227 = 0 ("DeviceIn")
            n129 = call "ATS_AsyncDMA_Device.vi"("DeviceIn"=w227, "ATS_Async_Ctrl"=ATS_Async_Ctrl."Stop") -> ("ReadSamples_Out"=w226:T37)  [unwired: 9 in, 4 out]
            n130 = call "ATS_AsyncDMA_Device.vi"("DeviceIn"=w227, "ATS_Async_Ctrl"=ATS_Async_Ctrl."Abort", "ReadSamples"=w226) -> ()  [unwired: 8 in, 5 out]
          }
        }
      }
      frame "Save Sweep" {
        # "Gage if you need\nthe gage card,\nenable here"
        n131 = case shown="True" TRUE {
          tunnel: w231 -> [_ w233]
          frame False {
          }
          frame True {
            w237 = 0 ("DeviceIn")
            n132 = local read "Clock Length"() -> (w239:u32)
            n133 = local read "Async_Setting"() -> (w235:T1)
            n134 = Bundle By Name(cluster=w235, "UseHeader"=u32 0, "Rec/Buffer"=u32 125, "Total_Rec"=u32 0) -> (w236:T1)
            n135 = Unbundle By Name(w233) -> ("Record.Presize"=w240:u32)
            n136 = Bundle By Name(cluster=T37 {"Offset"=0, "Length"=0} ("ReadSamples"), "Length"=w239, "Offset"=w240) -> (w238:T37)
            n137 = call "ATS_AsyncDMA_Device.vi"("DeviceIn"=w237, "ATS_Async_Ctrl"=ATS_Async_Ctrl."SetupDMA" ("ATS_DMA_Ctrl"), "Async_Mode"=ATS_Async_Mode."Traditional", "Async_Setting"=w236, "Channel"=ATS_DMA_Channel."Channel_B", "ReadSamples"=w238, "Start Now / Wait"=TRUE) -> ("Buffer"=w245:u16[])  [unwired: 4 in, 4 out]
            n138 = while {
              tunnel: w245 -> [_]
              shift-right: [ATS_Async_Ctrl."Get" ("ATS_Async_Ctrl")] -> _
              shift-left: ATS_Async_Ctrl."StartCapture" ("ATS_Async_Ctrl") -> [w259]
              tunnel: w237 -> [w253]
              stop <- w256 stop-if-true
              n139 = call "ATS_AsyncDMA_Device.vi"("DeviceIn"=w253, "ATS_Async_Ctrl"=w259) -> ("Buffer"=w251:u16[], "Async_Status"=w250:T5)  [unwired: 9 in, 3 out]
              n140 = Unbundle By Name(w250) -> ("Valid"=w252:bool, "Completed"=w261:bool, "Start DMA"=w262:bool, "Timeout"=w263:bool, "Error"=w260:bool)
              n141 = property on="Reset DAQ" class="Bool (strict)"() -> ("Value"=w257:bool)  [unwired: 2 in, 2 out]
              n142 = local read "Clock Length"() -> (w254:u32)
              n143 = Compound Arithmetic op=OR(w261, invert w262, w263, w260, w257) -> (w255:bool)
              n144 = case shown="True" w252 {
                selector: w252 -> [w264 w267]
                tunnel: w251 -> [_ w266]
                tunnel: [w264 w267] -> w256
                tunnel: w255 -> [_ _]
                tunnel: w254 -> [_ w265]
                frame False {
                }
                frame True {
                  n145 = Array Subset(array=w266, length=w265) -> (w268:u16[])  [unwired: 1 in]
                  n146 = call "Clock Frequency generator hilbert.vi"(7:6300.0 ("Sweep Speed"), "Acquisition speed (S/s)"=180000000.0 ("Sweep Speed"), "k-space signal in"=w268, "number of frequency updates"=4385) -> ("Error Out"=w273:errorcluster, "frequency\nsteps"=w272:i32)  [unwired: 6 in]
                  n147 = call "wavepond sequence.vi"("Error In"=w273, "Number of updates"=w272) -> ()  [unwired: 9 in, 1 out]
                }
              }
            }
          }
        }
      }
      frame "Initialize DAQ" {
        # "B-Scans per buffer should be around 4 if \ntaking more than 1 to minimize data transfer"
        # "If B Scans is 1, set total records to 0,\notherwise it should be A-Scans Per\nBScan times BScans"
        # "BScans Per Buffer"
        n148 = local read "First Time?"() -> (w278:bool)
        n149 = case shown="False" w278 {
          tunnel: [_ w310] -> w304
          tunnel: w281 -> [_ w306]
          tunnel: [FALSE ("First Time?") FALSE ("First Time?")] -> w277
          frame False {
          }
          frame True {
            n150 = call "ATS_Device.vi"("BoardToVerify"=w306, "ATS_Check"=ATS_Check_Ctrl."Verify Board", "DevCtrl"=Device_Ctrl."Initialize", "DeviceIn"=0 ("Device")) -> ("error out"=w308:errorcluster, "DeviceOut"=w312:i32)  [unwired: 1 in, 5 out]
            n151 = call "ATS_Device.vi"("error in (no error)"=w308, "DevCtrl"=Device_Ctrl."Abort", "DeviceIn"=w312) -> ("DeviceOut"=w310:i32)  [unwired: 2 in, 6 out]
          }
        }
        n152 = local write "First Time?"(w277) -> ()
        n153 = Unbundle By Name(w274) -> ("Record.Length"=w282:u32)
        n154 = call "ATS_MS_Set_Device.vi"("Set_Manually (F)"=FALSE, "Setup_In"=w274, "DeviceIn"=w304) -> ("Setup_Out"=w275:T7)  [unwired: 3 in, 5 out]
        n155 = local read "Scanning"() -> (w300:T26)
        n156 = Unbundle By Name(w300) -> ("B-scans (rings)"=w288:u32, "A(cluster)/B"=w298:u32, "B-scans (rings)"=w293:u32, "A(cluster)/B"=w292:u32, "B-scans (rings)"=w290:u32, "A(cluster)/B"=w284:u32)
        n157 = Not Equal?(x=w290, y=u32 1 ("x")) -> (x != y?=w291:bool)
        n158 = Equal?(x=u32 1, y=w288) -> (x = y?=w294:bool)
        n159 = local read "B-Scans Per Buffer"() -> (w276:i32)
        n160 = Select(t=u32 4 ("y"), s=w294, f=w276) -> (s? t:f=w296:u32)
        n161 = Multiply(x=w293, y=w292) -> (x*y=w287:u32)
        n162 = local read "Async_Setting"() -> (w280:T1)
        n163 = Select(t=w287, s=w291, f=u32 0 ("Total_Rec")) -> (s? t:f=w302:u32)
        n164 = Multiply(x=w296, y=w298) -> (x*y=w299:u32)
        n165 = Bundle By Name(cluster=T6 {"Points Per A-Scan"=0, "A-Scans per B-Scan"=0, "Voltage Range"=4.0, "Card Resolution (bits)"=16} ("Imaging Parameters"), "Points Per A-Scan"=w282, "A-Scans per B-Scan"=w284) -> (w283:T6)
        n166 = Bundle By Name(cluster=w280, "UseHeader"=u32 0, "Rec/Buffer"=w299, "Total_Rec"=w302) -> (w279:T1)
        n167 = local write "Async_Setting"(w279) -> ()
        n168 = local write "Imaging Parameters"(w283) -> ()
      }
      frame "Acquire Data", Default {
        w337 = 0 ("DeviceIn")
        # "Update and \nclear the \nEn Face"
        # "Tell the FFT the most\nup-to-date imaging\nparameters"
        n169 = Enqueue Element(queue=w329, element=OCT_Hardware_States."Stop", error in (no error)=w320) -> (error out=w319:errorcluster)  [unwired: 1 in, 2 out]
        n170 = local read "Imaging Parameters"() -> (w326:T6)
        n171 = local read "Data Format"() -> (w331:T23)
        n172 = local read "Async_Setting"() -> (w324:T1)
        n173 = case shown="\"Channel 1\", Default" w331 {
          tunnel: [ATS_DMA_Channel."Channel_A" ("Channel") ATS_DMA_Channel."A & B" ("Channel") ATS_DMA_Channel."A & B" ("Channel")] -> w330
          frame "Channel 1", Default {
          }
          frame "Channel 2" {
          }
          frame "Channel 1 and 2" {
          }
        }
        n174 = call "OCT Processing 2ch functional global.vi"("State"=processing_states."Update Imaging Parameters", "error in (no error)"=w319, "Input Parameters"=w326) -> ("error out"=w328:errorcluster)  [unwired: 4 in, 4 out]
        n175 = local read "Scanning"() -> (w323:T26)
        n176 = call "En Face Functional Global.vi"(7:En_Face_States."Clear En Face" ("En Face States"), "Error In"=w328, 9:w323) -> ("Error Out"=w322:errorcluster)  [unwired: 7 in, 1 out]
        n177 = Unbundle By Name(w316) -> ("Record.Length"=w333:u32, "Record.Presize"=w332:u32)
        n178 = Unbundle By Name(w316) -> ("Record.Length"=w315:u32)
        n179 = call "OCT Processing 2ch functional global.vi"("State"=processing_states."Get Queue", "error in (no error)"=w322) -> ("queue out"=w318:refnum<queue>)  [unwired: 5 in, 4 out]
        n180 = Bundle By Name(cluster=T37 {"Offset"=0, "Length"=0} ("ReadSamples"), "Length"=w333, "Offset"=w332) -> (w339:T37)
        n181 = call "ATS_AsyncDMA_Device.vi"("DeviceIn"=w337, "ATS_Async_Ctrl"=ATS_Async_Ctrl."SetupDMA" ("ATS_DMA_Ctrl"), "Async_Mode"=ATS_Async_Mode."No-Pre-Trigger", "Async_Setting"=w324, "Channel"=w330, "ReadSamples"=w339, "Start Now / Wait"=TRUE) -> ("Buffer"=w335:u16[])  [unwired: 4 in, 4 out]
        n182 = while {
          tunnel: w335 -> [_]
          tunnel: w337 -> [w363]
          shift-right: [ATS_Async_Ctrl."Get" ("ATS_Async_Ctrl")] -> _
          shift-left: ATS_Async_Ctrl."StartCapture" ("ATS_Async_Ctrl") -> [w360]
          tunnel: w318 -> [w352]
          tunnel: [w351] -> w317
          tunnel: w315 -> [w350]
          stop <- w351 stop-if-true
          n183 = call "ATS_AsyncDMA_Device.vi"("DeviceIn"=w363, "ATS_Async_Ctrl"=w360) -> ("Buffer"=w356:u16[], "Async_Status"=w358:T5)  [unwired: 9 in, 3 out]
          "Async_Status" <- w358
          n184 = Unbundle By Name(w358) -> ("Valid"=w357:bool, "Completed"=w353:bool, "Start DMA"=w354:bool, "Timeout"=w362:bool, "Error"=w361:bool)
          n185 = local read "Reset DAQ"() -> (w355:bool)
          n186 = Compound Arithmetic op=OR(w353, invert w354, w362, w361, w355) -> (w351:bool)
          n187 = case shown="True" w357 {
            tunnel: w356 -> [_ w368]
            tunnel: w352 -> [_ w370]
            tunnel: w350 -> [_ w367]
            frame False {
              # "Do nothing"
            }
            frame True {
              n188 = Enqueue Element(queue=w370, element=w368, timeout in ms (-1)=50) -> (error out=w365:errorcluster)  [unwired: 1 in, 2 out]
              n189 = property on="Save Sweep" class="Bool"(error in=w365, "DisabledEnum"=T35."Enabled" ("Disabled")) -> ()  [unwired: 1 in, 2 out]
              n190 = call "Display Raw Data.vi"("Enum"=Display_Raw_Data_states."Add Processed", "Length"=w367, "Raw Data In"=w368) -> ()  [unwired: 9 in]
            }
          }
        }
        n191 = while {
          tunnel: w317 -> [w346]
          stop <- w344 stop-if-true
          n192 = local read "Processing Finished"() -> (w345:bool)
          n193 = Wait (ms)(milliseconds to wait=u32 50) -> ()  [unwired: 1 out]
          n194 = And(x=w346, y=w345) -> (x .and. y?=w344:bool)
        }
      }
      frame "Acquire Data" {
        w399 = 0 ("DeviceIn")
        # "Close files and set save \nstate to do nothing"
        # "Update and \nclear the \nEn Face"
        # "Tell the FFT the most\nup-to-date imaging\nparameters"
        n195 = local read "Imaging Parameters"() -> (w388:T6)
        n196 = local read "Data Format"() -> (w393:T23)
        n197 = local read "Async_Setting"() -> (w384:T1)
        n198 = case shown="\"Channel 1\", Default" w393 {
          tunnel: [ATS_DMA_Channel."Channel_A" ("Channel") ATS_DMA_Channel."A & B" ("Channel") ATS_DMA_Channel."A & B" ("Channel")] -> w392
          frame "Channel 1", Default {
          }
          frame "Channel 2" {
          }
          frame "Channel 1 and 2" {
          }
        }
        n199 = call "OCT Processing 2ch functional global.vi"("State"=processing_states."Update Imaging Parameters", "error in (no error)"=w376, "Input Parameters"=w388) -> ("error out"=w390:errorcluster)  [unwired: 4 in, 4 out]
        n200 = local read "Scanning"() -> (w383:T26)
        n201 = call "En Face Functional Global.vi"(7:En_Face_States."Clear En Face" ("En Face States"), "Error In"=w390, 9:w383) -> ("Error Out"=w382:errorcluster)  [unwired: 7 in, 1 out]
        n202 = Unbundle By Name(w374) -> ("Record.Length"=w395:u32, "Record.Presize"=w394:u32)
        n203 = call "Save Data Functional Global.vi"("States"=Saving_Data_States."Get Queue", "error in (no error)"=w376) -> ("Saving Queue Out"=w377:refnum<queue>)  [unwired: 6 in, 3 out]
        n204 = call "OCT Processing 2ch functional global.vi"("State"=processing_states."Get Queue", "error in (no error)"=w382) -> ("error out"=w381:errorcluster, "queue out"=w379:refnum<queue>)  [unwired: 5 in, 3 out]
        n205 = Bundle By Name(cluster=T37 {"Offset"=0, "Length"=0} ("ReadSamples"), "Length"=w395, "Offset"=w394) -> (w401:T37)
        n206 = call "ATS_AsyncDMA_Device.vi"("DeviceIn"=w399, "ATS_Async_Ctrl"=ATS_Async_Ctrl."SetupDMA" ("ATS_DMA_Ctrl"), "Async_Mode"=ATS_Async_Mode."No-Pre-Trigger", "Async_Setting"=w384, "Channel"=w392, "ReadSamples"=w401, "Start Now / Wait"=TRUE) -> ("Buffer"=w397:u16[])  [unwired: 4 in, 4 out]
        n207 = while {
          tunnel: w381 -> [_]
          tunnel: [w412] -> w387
          tunnel: [w410] -> w372
          i -> [w411]
          stop <- w410 stop-if-true
          # "Saves data as long as data is being fed into the Queue,\notherwise it will time out and halt this loop."
          n208 = case shown="1, Default" w411 {
            tunnel: [FALSE w415] -> w410
            tunnel: [_ w416] -> w412
            frame 0 {
              # "Wait for data to Q up"
              n209 = Wait (ms)(milliseconds to wait=u32 1000) -> ()  [unwired: 1 out]
            }
            frame 1, Default {
              n210 = local read "Data Format"() -> (w418:T23)
              n211 = call "Save Data Functional Global.vi"("States"=Saving_Data_States."Save Data", "Data Format"=w418) -> ("error out"=w416:errorcluster, "Time Out"=w415:bool)  [unwired: 6 in, 2 out]
            }
          }
        }
        n212 = while {
          tunnel: w397 -> [_]
          tunnel: w399 -> [w432]
          shift-right: [ATS_Async_Ctrl."Get" ("ATS_Async_Ctrl")] -> _
          shift-left: ATS_Async_Ctrl."StartCapture" ("ATS_Async_Ctrl") -> [w429]
          tunnel: w379 -> [w421]
          tunnel: w377 -> [w420]
          tunnel: [w419] -> w373
          stop <- w419 stop-if-true
          n213 = call "ATS_AsyncDMA_Device.vi"("DeviceIn"=w432, "ATS_Async_Ctrl"=w429) -> ("Buffer"=w425:u16[], "Async_Status"=w427:T5)  [unwired: 9 in, 3 out]
          n214 = Unbundle By Name(w427) -> ("Valid"=w426:bool, "Completed"=w422:bool, "Start DMA"=w423:bool, "Timeout"=w431:bool, "Error"=w430:bool)
          n215 = local read "Reset DAQ"() -> (w424:bool)
          n216 = Compound Arithmetic op=OR(w422, invert w423, w431, w430, w424) -> (w419:bool)
          n217 = case shown="True" w426 {
            tunnel: w425 -> [_ w435]
            tunnel: w425 -> [_ w436]
            tunnel: w421 -> [_ w437]
            tunnel: w420 -> [_ w434]
            frame False {
              # "Do nothing"
            }
            frame True {
              w433 = 50 ("timeout in ms (-1)")
              n218 = Enqueue Element(queue=w434, element=w435, timeout in ms (-1)=w433) -> ()  [unwired: 1 in, 3 out]
              n219 = Enqueue Element(queue=w437, element=w436, timeout in ms (-1)=w433) -> ()  [unwired: 1 in, 3 out]
            }
          }
        }
        n220 = call "Save Data Functional Global.vi"("States"=Saving_Data_States."Close Files", "error in (no error)"=w387) -> ("error out"=w386:errorcluster)  [unwired: 6 in, 3 out]
        n221 = call "Save Data Functional Global.vi"("States"=Saving_Data_States."Do Nothing" ("Save State"), "error in (no error)"=w386) -> ()  [unwired: 6 in, 4 out]
        n222 = And(x=w373, y=w372) -> (x .and. y?=w371:bool)
        n223 = flat-sequence {
          tunnel: w391 -> [w406]
          tunnel: w371 -> [_]
          frame #0 {
            n224 = Enqueue Element(queue=w406, element=OCT_Hardware_States."Stop") -> ()  [unwired: 2 in, 3 out]
          }
        }
      }
      frame "Set Resampling Array" {
        n225 = Wait (ms)(milliseconds to wait=u32 10) -> ()  [unwired: 1 out]
      }
      frame "Stop" {
        n226 = Release Queue(queue=w449, error in (no error)=w448) -> (error out=w447:errorcluster)  [unwired: 1 in, 2 out]
        n227 = call "OCT Processing 2ch functional global.vi"("State"=processing_states."Shutdown", "error in (no error)"=w447) -> ("error out"=w446:errorcluster)  [unwired: 5 in, 4 out]
        n228 = call "Save Data Functional Global.vi"("States"=Saving_Data_States."Shutdown", "error in (no error)"=w446) -> ("error out"=w443:errorcluster)  [unwired: 6 in, 3 out]
        n229 = call "galvo_functional_global.vi"("State"=galvo_states."Shutdown", "error in (no error)"=w443) -> ("error out"=w442:errorcluster)  [unwired: 8 in, 1 out]
        n230 = flat-sequence {
          tunnel: w442 -> [_]
          frame #0 {
            w453 = 0 ("DeviceIn")
            n231 = call "ATS_AsyncDMA_Device.vi"("DeviceIn"=w453, "ATS_Async_Ctrl"=ATS_Async_Ctrl."Stop") -> ("ReadSamples_Out"=w452:T37)  [unwired: 9 in, 4 out]
            n232 = call "ATS_AsyncDMA_Device.vi"("DeviceIn"=w453, "ATS_Async_Ctrl"=ATS_Async_Ctrl."Abort", "ReadSamples"=w452) -> ()  [unwired: 8 in, 5 out]
          }
          frame #1 {
            n233 = Stop(stop? (T)=TRUE) -> ()
          }
        }
      }
      frame "Set Clock" {
        w458 = T15 12 items=["20mV", "40mV", "50mV", "80mV", "100mV", "200mV", "400mV", "500mV", "800mV", "1 V", "1.25 V", "2 V", "4 V", "5 V", "8 V", "10 V", "16 V", "20 V", "40 V", "HiFi"] ("Input B.Range")
        w461 = u32 18 items=["1 kS/s", "2 kS/s", "5 kS/s", "10 kS/s", "20 kS/s", "50 kS/s", "100 kS/s", "200 kS/s", "500 kS/s", "1 MS/s", "2 MS/s", "5 MS/s", "10 MS/s", "20 MS/s", "50 MS/s", "100 MS/s", "125 MS/s", "160 MS/s", "180 MS/s"] ("ClckRate")
        n234 = local read "Clock Length"() -> (w460:u32)
        n235 = call "ATS_Device.vi"("BoardToVerify"=w456, "ATS_Check"=ATS_Check_Ctrl."Verify Board", "DevCtrl"=Device_Ctrl."Initialize", "DeviceIn"=0 ("Device")) -> ("error out"=w463:errorcluster, "DeviceOut"=w468:i32)  [unwired: 1 in, 5 out]
        n236 = Bundle By Name(cluster=w455, "Record.Length"=w460, "Clock.ClckSource"=ClockSource."Internal", "Clock.ClckRate"=w461, "Input B.Range"=w458, "Input A.Impedance"=Impedance."50 ohms") -> (w459:T7)
        n237 = call "ATS_Device.vi"("error in (no error)"=w463, "DevCtrl"=Device_Ctrl."Abort", "DeviceIn"=w468) -> ("DeviceOut"=w466:i32)  [unwired: 2 in, 6 out]
        n238 = call "ATS_MS_Set_Device.vi"("Set_Manually (F)"=FALSE, "Setup_In"=w459, "DeviceIn"=w466) -> ()  [unwired: 3 in, 6 out]
      }
    }
  }
  n239 = Destroy User Event(user event=w6) -> ()  [unwired: 1 in, 1 out]
